vi "AnalogDemultiplexerV2_NI5771.vi"() -> ()   [LabVIEW 2012]
uses:
  <vilib>/Platform/TimedLoop/XDataNode/timing_clust.ctl
  <vilib>/Platform/TimedLoop/XDataNode/nitl_modes.ctl
  <vilib>/Platform/TimedLoop/XDataNode/wakeup.ctl
  <vilib>/rvi/FIFO/Fifo_Resource/nirvififoEmulationSetSize.vi
  <vilib>/rvi/DataTransferAndStorage/Container/Common/niFpgaContainerGetUniqueNameForEmu.vi
  <vilib>/rvi/eio/common/nirviEmuTemplateMethod_errors.vi
  <vilib>/rvi/Emulation/niFpgaSctlEmulationRegisterWithScheduler.vi
  <vilib>/rvi/errors/niFpgaSetErrorForExecOnDevCompSimple.vi
  <vilib>/rvi/eio/common/nirviEmuReportErrorAndStop.vi
  <vilib>/rvi/Emulation/niFpgaSctlEmulationFifoFullMgr.vi
  <vilib>/rvi/Emulation/niFpgaSctlEmulationResourceMgr.vi
  <vilib>/rvi/Emulation/niFpgaSctlEmulationScheduler.vi
  <vilib>/rvi/interface/RandomDataEmulation/nirviRandomDataFPGAFIFO.vi
  <vilib>/rvi/interface/RandomDataEmulation/niFpgaRandomDataHandleErrors.vi
  <vilib>/rvi/Emulation/niFpgaSctlEmulationGlobalWrite.vi
  <vilib>/Platform/TimedLoop/XDataNode/XDataNode.xnode
  <vilib>/rvi/DataTransferAndStorage/Container/XNode/niFpgaContainer.xnode
  <vilib>/rvi/FIFO/Fifo_Resource/nirvififoEmulationClear.vi
  <vilib>/eio/EIONode/EIONode.xnode
  <vilib>/rvi/FIFO/Fifo_Resource/nirvififoEmulationWrite.vi
  <vilib>/rvi/FIFO/Fifo_Resource/nirvififoEmulationRead.vi
  <vilib>/rvi/interface/RandomDataEmulation/nirviRandomDataFpgaReadWriteTemplate.vi
  <vilib>/Platform/TimedLoop/XDataNode/XDNodeRunTimeDep.lvlib
panel:
  in  "CutoffU8 Ch2":u8
  in  "CutoffU8 Ch1":u8
  out "ToHostA2FIFO Overflow":bool
  out "ToHostA1FIFO Overflow":bool
  out "Pixel counter A2":u32
  out "Pixel counter A1":u32
  out "InterloopFIFO Overflow":bool
  in  "BaselineU8 Ch2":u8
  in  "BaselineU8 Ch1":u8
  out "InterloopFIFO timeout":bool
  in  "Clear Interloop FIFO":bool
  out "Acquiring":bool
  in  "Wait for trigger":bool
  in  "Acquire":bool
  in  "Requested pixels A2":u32=100000 caption="Requested pixels"
  in  "Acquire continuously":bool=TRUE
  in  "Requested pixels A1":u32=100000 caption="Requested pixels"
  in  "Samples per pixel":u16=10000 caption="Samples per pixel Acq"
  out "IO Module\\AI Over Range":bool
  in  "User Command Commit":bool
  in  "User Command":u8
  out "User Command Idle":bool
  out "User Command Status":u8
  in  "User Data 0":u16
  in  "User Data 1":u8
  out "PLL Locked":bool
  out "User Error":bool
  out "Configured?":bool
  # "5771 IO module configuration"
  # "Analog demultiplexer V2"
  # "Acquisition control"
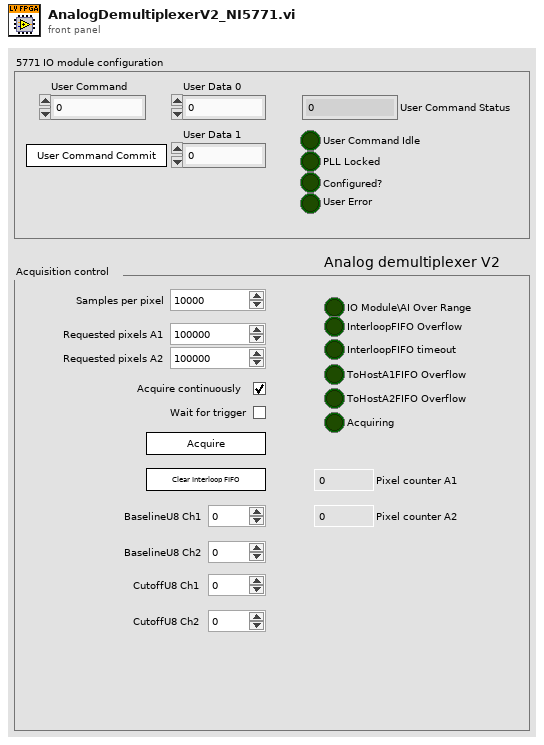
[diagram p1: front panel]
types:
  T1 = typedef "XDNodeRunTimeDep.lvlib/timing_clust.ctl" = cluster{"Expected End [f-1]":u64, "Actual End [f-1]":u64, "Finished Late? [f-1]":bool, "Expected End [i-1]":u64, "Actual End [i-1]":u64, "Finished Late? [i-1]":bool, "Expected Start [i]":u64, "Actual Start [i]":u64, "Expected Start [f]":u64, "Actual Start [f]":u64, "Source Name":string, "Structure Name":string, "Period":i64, "Deadline":i64, "Offset":i64, "Start":i64, "Priority":i32, "Timeout":i32, "Mode":T2, "Wakeup Reason":T3, "Error":errorcluster, "Source Type":string, "Secondary Source Type":string, "Global End Time":u64, "Global Start Time":u64, "Frame Duration":u64, "Iteration Duration":u64, "Assigned CPU":i32, "I/O Scan Engine Mode":u32}
  T2 = typedef "XDNodeRunTimeDep.lvlib/nitl_modes.ctl" = enum32{"No Change", "Process missed periods, maintain original phase", "Discard missed periods, maintain original phase", "Process missed periods, ignore original phase", "Discard missed periods, ignore original phase"}
  T3 = typedef "XDNodeRunTimeDep.lvlib/wakeup.ctl" = enum32{"Normal", "Aborted", "Asynchronous wakeup", "Timing source error", "Timed loop error", "Timeout"}
  T4 = cluster{"IO Module\\AI 0 Data N-7":u8, "IO Module\\AI 0 Data N-6":u8, "IO Module\\AI 0 Data N-5":u8, "IO Module\\AI 0 Data N-4":u8, "IO Module\\AI 0 Data N-3":u8, "IO Module\\AI 0 Data N-2":u8, "IO Module\\AI 0 Data N-1":u8, "IO Module\\AI 0 Data N":u8, "IO Module\\Synchronous Trigger Input":u8}
  T5 = cluster{"IO Module\\AI 1 Data N-7":u8, "IO Module\\AI 1 Data N-6":u8, "IO Module\\AI 1 Data N-5":u8, "IO Module\\AI 1 Data N-4":u8, "IO Module\\AI 1 Data N-3":u8, "IO Module\\AI 1 Data N-2":u8, "IO Module\\AI 1 Data N-1":u8, "IO Module\\AI 1 Data N":u8, "IO Module\\Synchronous Trigger Input":u8}
  T6 = cluster{"A1 Ch1":u32, "A1 Ch2":u32, "A2 Ch1":u32, "A2 Ch2":u32}
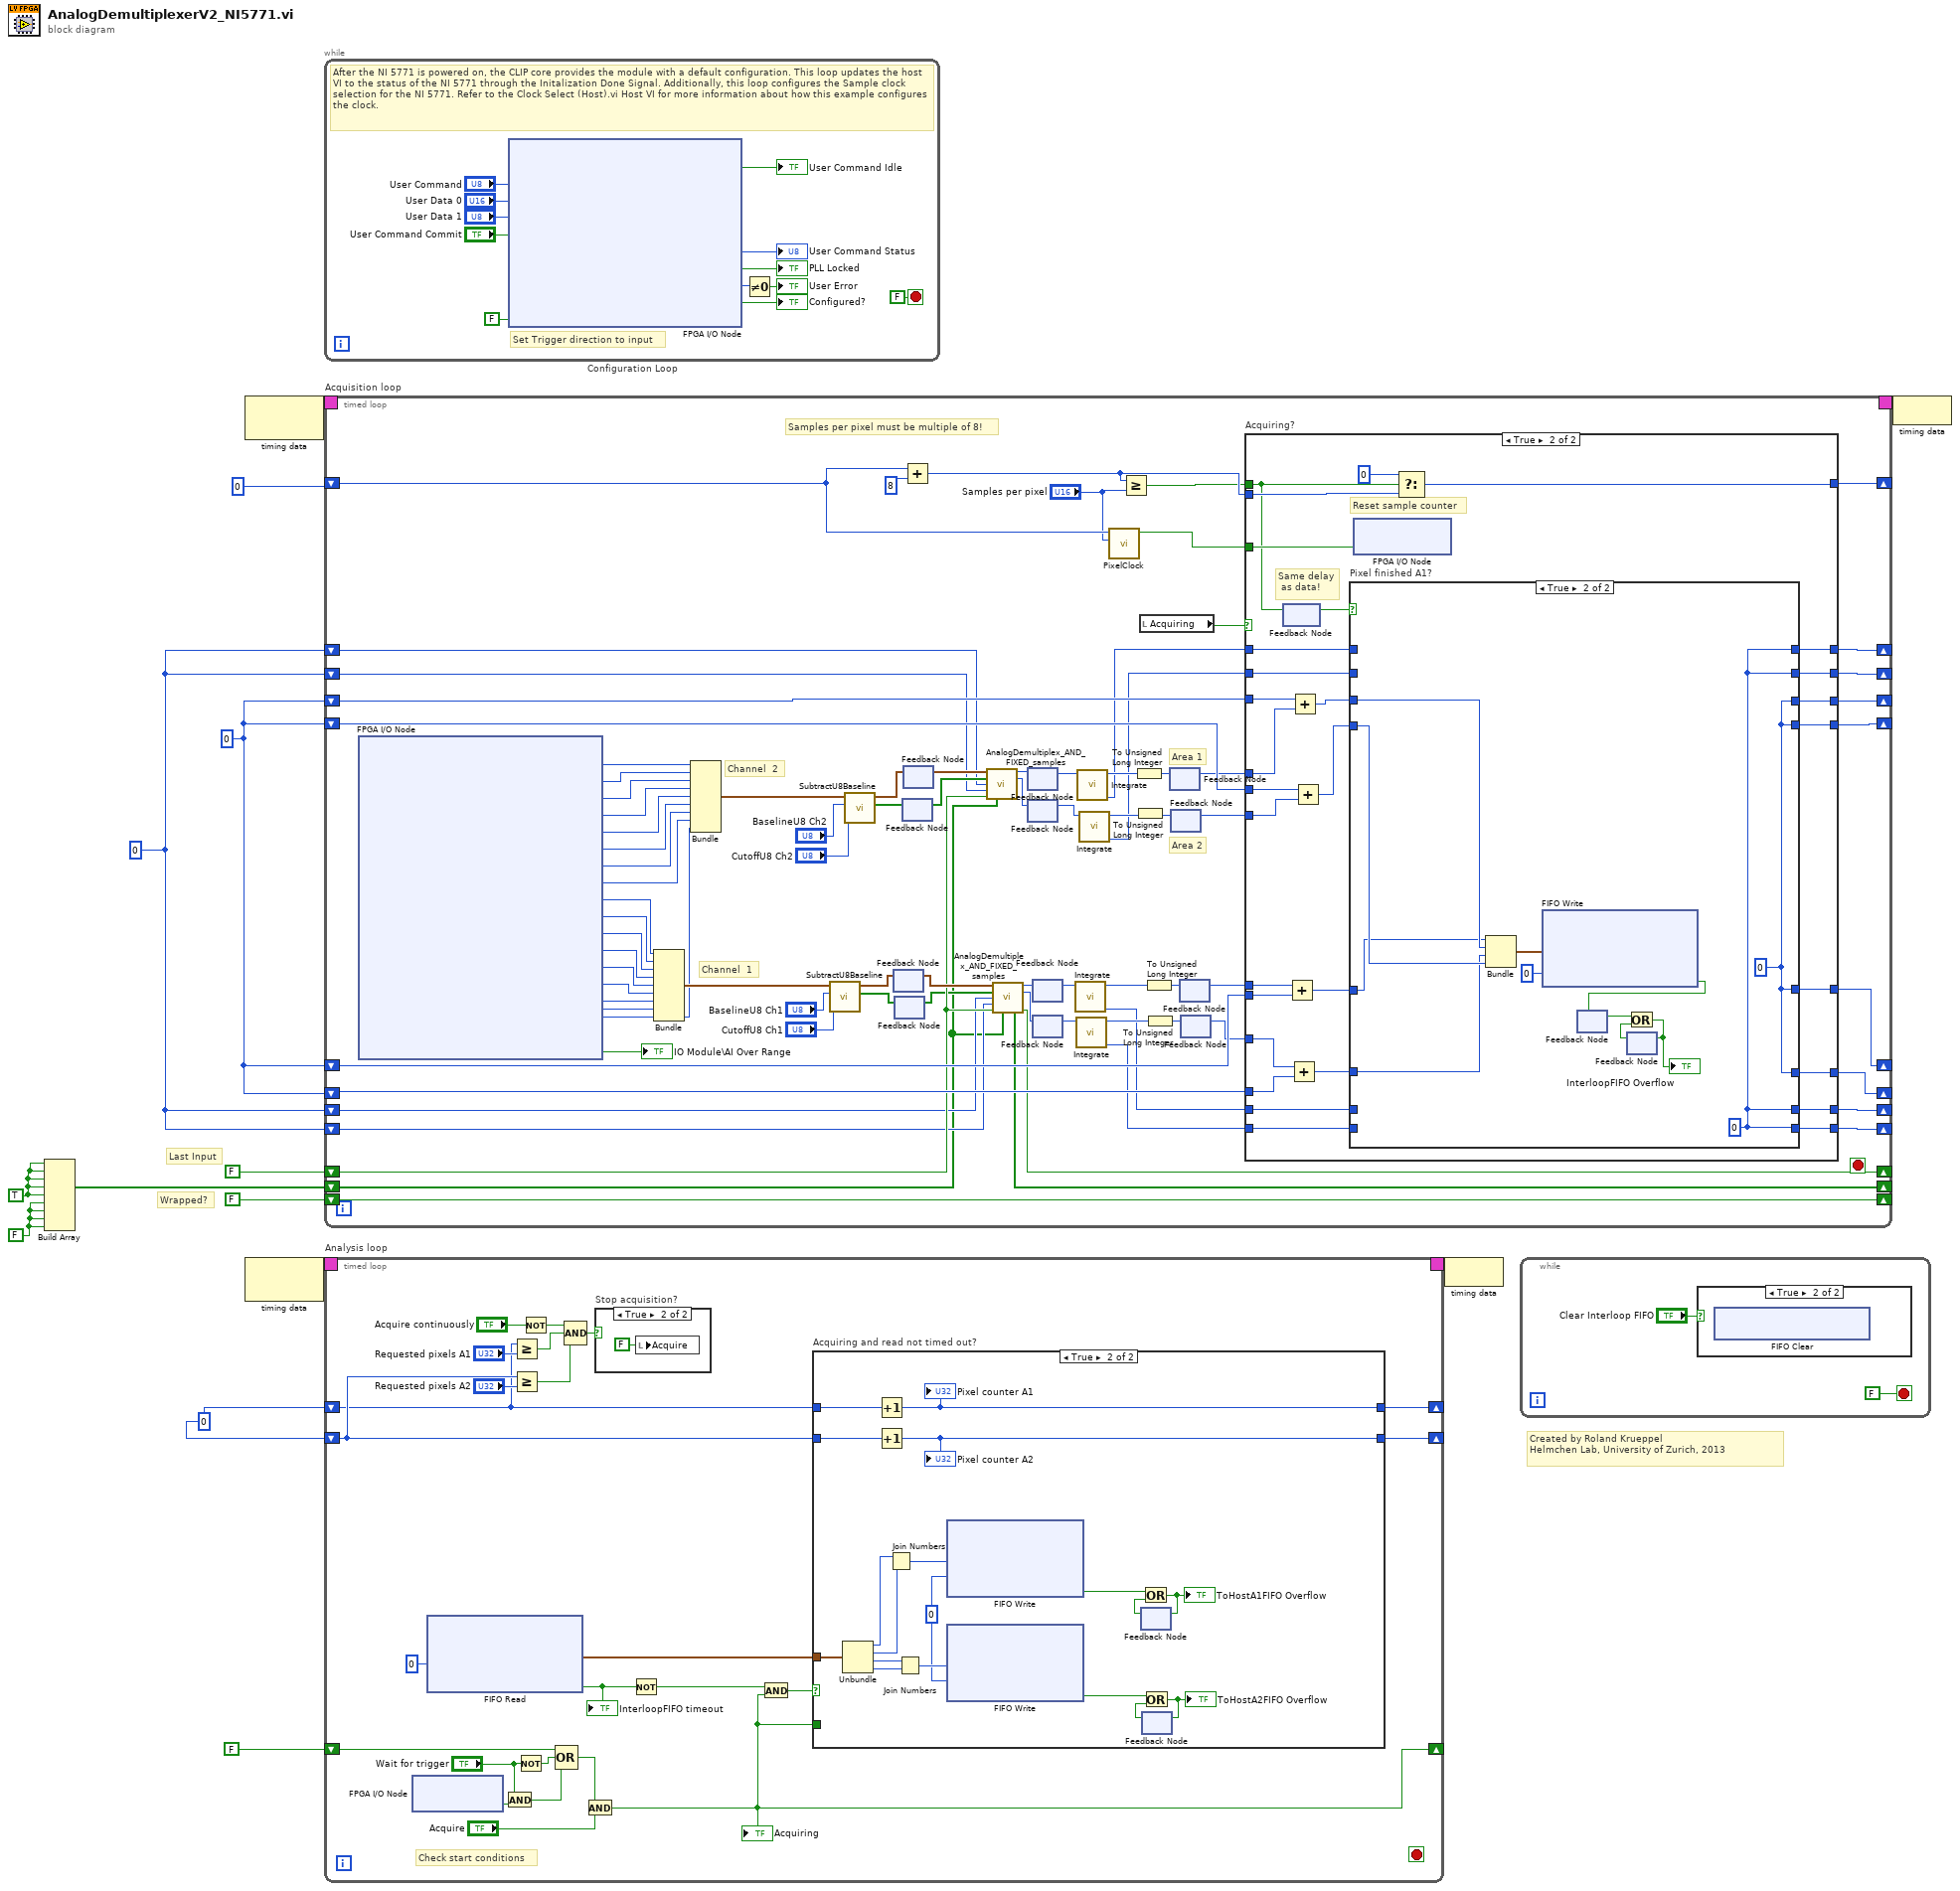
[diagram p0: block diagram]
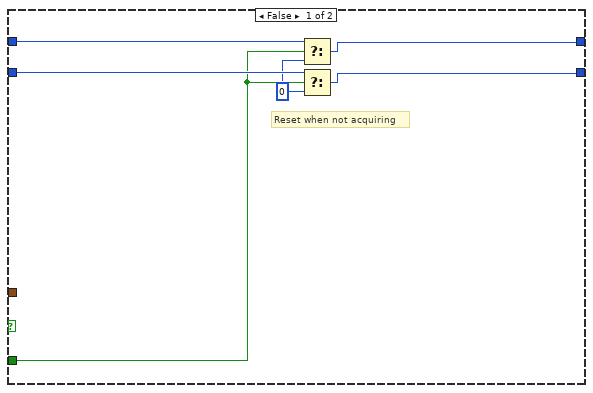
[diagram p3: hidden frame]
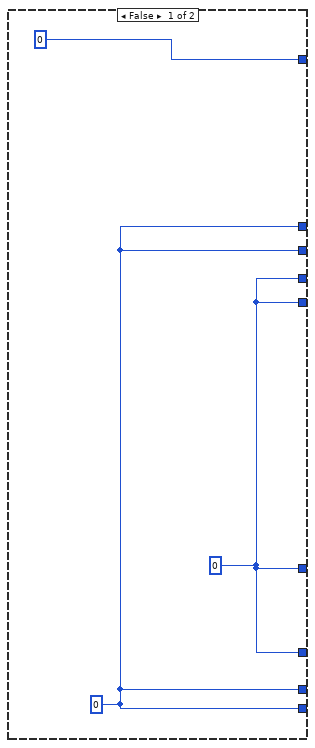
[diagram p5: hidden frame]
diagram:
  w1 = FALSE
  w2 = TRUE
  w4 = u8 0
  w6 = u32 0
  w9 = u32 0 ("Integrator out")
  # "Wrapped?"
  # "Last Input"
  # "Created by Roland Krueppel\nHelmchen Lab, University of Zurich, 2013"
  n1 = Build Array(w2, w2, w2, w2, w2, w1, w1, w1, w1) -> (w3:bool[])
  n2 = node-c288() -> (w14:T1)  [unwired: 1 in]
  n3 = node-c288() -> (w12:T1)  [unwired: 1 in]
  n4 = while "Configuration Loop" {
    stop <- FALSE stop-if-true
    # "Set Trigger direction to input"
    # "After the NI 5771 is powered on, the CLIP core provides the module with a default configuration. This loop updates the host VI to the status of the NI 5771 through the Initalization Done Signal. Additionally, this loop configures the Sample clock selection for the NI 5771. Refer to the Clock Select (Host).vi Host VI for more information about how this example configures the clock."
    n5 = xnode "FPGA I/O Node"("IO Module\\User Command"="User Command", "IO Module\\User Data 0"="User Data 0", "IO Module\\User Data 1"="User Data 1", "IO Module\\User Command Commit"="User Command Commit", "IO Module\\Trigger WE"=FALSE ("IO Module\\Trigger WE")) -> ("IO Module\\User Command Idle"=→"User Command Idle":bool, "IO Module\\User Command Status"=→"User Command Status":u8, "IO Module\\PLL Locked"=→"PLL Locked":bool, "IO Module\\User Error"=w19:u8, "IO Module\\Initialization Done"=→"Configured?":bool)  [unwired: 10 in, 10 out]
    n6 = Not Equal To 0?(x=w19) -> (x != 0?=→"User Error":bool)
  }
  n7 = timed-loop "Acquisition loop" {
    timing: w14 -> [_]
    timing-out: [_] -> w13
    shift-right: [w95] -> _
    shift-left: u16 0 -> [w86]
    shift-right: [w68] -> _
    shift-left: w6 -> [w77]
    shift-right: [w67] -> _
    shift-left: w6 -> [w76]
    shift-right: [w69] -> _
    shift-left: w6 -> [w78]
    shift-right: [w70] -> _
    shift-left: w6 -> [w79]
    shift-right: [w41] -> _
    shift-left: FALSE -> [w51]
    shift-right: [w56] -> _
    shift-left: FALSE -> [w56]
    shift-right: [w48] -> _
    shift-left: w4 -> [w30]
    shift-right: [w47] -> _
    shift-left: w4 -> [w29]
    shift-right: [w50] -> _
    shift-left: w4 -> [w31]
    shift-right: [w49] -> _
    shift-left: w4 -> [w32]
    shift-right: [w28] -> _
    shift-left: w3 -> [w27]
    stop <- _ stop-if-true
    # "Area 2"
    # "Area 1"
    # "Channel  2"
    # "Channel  1"
    # "Samples per pixel must be multiple of 8!"
    n8 = xnode "FPGA I/O Node"() -> ("IO Module\\AI 1 Data N-7"=w103:u8, "IO Module\\AI 1 Data N-6"=w102:u8, "IO Module\\AI 1 Data N-5"=w101:u8, "IO Module\\AI 1 Data N-4"=w100:u8, "IO Module\\AI 1 Data N-3"=w99:u8, "IO Module\\AI 1 Data N-2"=w98:u8, "IO Module\\AI 1 Data N-1"=w97:u8, "IO Module\\AI 1 Data N"=w96:u8, "IO Module\\AI 0 Data N-7"=w104:u8, "IO Module\\AI 0 Data N-6"=w105:u8, "IO Module\\AI 0 Data N-5"=w106:u8, "IO Module\\AI 0 Data N-4"=w107:u8, "IO Module\\AI 0 Data N-3"=w108:u8, "IO Module\\AI 0 Data N-2"=w109:u8, "IO Module\\AI 0 Data N-1"=w110:u8, "IO Module\\AI 0 Data N"=w111:u8, "IO Module\\Synchronous Trigger Input"=w66:u8, "IO Module\\AI Over Range"=→"IO Module\\AI Over Range":bool)  [unwired: 18 in, 18 out]
    n9 = Bundle("IO Module\\AI 0 Data N-7"=w104, "IO Module\\AI 0 Data N-6"=w105, "IO Module\\AI 0 Data N-5"=w106, "IO Module\\AI 0 Data N-4"=w107, "IO Module\\AI 0 Data N-3"=w108, "IO Module\\AI 0 Data N-2"=w109, "IO Module\\AI 0 Data N-1"=w110, "IO Module\\AI 0 Data N"=w111, "IO Module\\Synchronous Trigger Input"=w66) -> (w89:T4)  [unwired: 1 in]
    n10 = Bundle("IO Module\\AI 1 Data N-7"=w103, "IO Module\\AI 1 Data N-6"=w102, "IO Module\\AI 1 Data N-5"=w101, "IO Module\\AI 1 Data N-4"=w100, "IO Module\\AI 1 Data N-3"=w99, "IO Module\\AI 1 Data N-2"=w98, "IO Module\\AI 1 Data N-1"=w97, "IO Module\\AI 1 Data N"=w96, "IO Module\\Synchronous Trigger Input"=w66) -> (w91:T5)  [unwired: 1 in]
    n11 = call "SubtractU8Baseline.vi"("Cutoff U8"="CutoffU8 Ch1", "Baseline U8"="BaselineU8 Ch1", "Analog data cluster in"=w89) -> ("Over? Array"=w38:bool[], "Analog data cluster out"=w88:T4)  [unwired: 7 in]
    n12 = call "SubtractU8Baseline.vi"("Cutoff U8"="CutoffU8 Ch2", "Baseline U8"="BaselineU8 Ch2", "Analog data cluster in"=w91) -> ("Over? Array"=w40:bool[], "Analog data cluster out"=w90:T4)  [unwired: 7 in]
    n13 = feedback #1() -> (w65:T4)  [unwired: 1 in]
    n14 = feedback-in #1(w88) -> ()
    n15 = feedback #2() -> (w37:bool[])  [unwired: 1 in]
    n16 = feedback-in #2(w38) -> ()
    n17 = Add(x=w86, y=u16 8) -> (x+y=w93:u16)
    n18 = feedback #3() -> (w39:bool[])  [unwired: 1 in]
    n19 = feedback-in #3(w40) -> ()
    n20 = feedback-in #4(w90) -> ()
    n21 = feedback #4() -> (w57:T4)  [unwired: 1 in]
    n22 = call "AnalogDemultiplex_AND_FIXED_samples.vi"("Analog data cluster"=w57, "Over? Array"=w39, "Last Sample A1"=w31, "Last Sample A2"=w32, "Last? Input"=w51, "array in"=w27) -> ("Data A1 out"=w61:u64, "Data A2 out"=w59:u64)  [unwired: 6 in, 2 out]
    n23 = call "AnalogDemultiplex_AND_FIXED_samples.vi"("Analog data cluster"=w65, "Over? Array"=w37, "Last Sample A1"=w30, "Last Sample A2"=w29, "Last? Input"=w51, "array in"=w27) -> ("Data A1 out"=w64:u64, "Data A2 out"=w63:u64, "array out"=w28:bool[], "Last? Output"=w41:bool)  [unwired: 6 in]
    n24 = feedback-in #5(w61) -> ()
    n25 = feedback #5() -> (w60:u64)  [unwired: 1 in]
    n26 = feedback #6() -> (w58:u64)  [unwired: 1 in]
    n27 = feedback-in #6(w59) -> ()
    n28 = feedback #7() -> (w84:u64)  [unwired: 1 in]
    n29 = feedback-in #7(w64) -> ()
    n30 = feedback #8() -> (w62:u64)  [unwired: 1 in]
    n31 = feedback-in #8(w63) -> ()
    n32 = call "Integrate.vi"("New samples in"=w84) -> ("Next Sample"=w43:u8, "Sum out"=w44:u16)  [unwired: 9 in]
    n33 = call "Integrate.vi"("New samples in"=w62) -> ("Next Sample"=w42:u8, "Sum out"=w45:u16)  [unwired: 9 in]
    n34 = call "Integrate.vi"("New samples in"=w60) -> ("Next Sample"=w33:u8, "Sum out"=w36:u16)  [unwired: 9 in]
    n35 = call "Integrate.vi"("New samples in"=w58) -> ("Next Sample"=w34:u8, "Sum out"=w35:u16)  [unwired: 9 in]
    n36 = call "PixelClock.vi"("Samples per pixel"="Samples per pixel", "Sample counter"=w86) -> ("Pixel clock"=w85:bool)  [unwired: 9 in]
    n37 = Greater Or Equal?(x=w93, y="Samples per pixel") -> (x >= y?=w92:bool)
    n38 = To Unsigned Long Integer(number=w36) -> (unsigned 32bit integer=w83:u32)
    n39 = To Unsigned Long Integer(number=w35) -> (unsigned 32bit integer=w82:u32)
    n40 = local read "Acquiring"() -> (w71:bool)
    n41 = To Unsigned Long Integer(number=w44) -> (unsigned 32bit integer=w81:u32)
    n42 = To Unsigned Long Integer(number=w45) -> (unsigned 32bit integer=w80:u32)
    n43 = feedback #9() -> (w74:u32)  [unwired: 1 in]
    n44 = feedback-in #9(w83) -> ()
    n45 = feedback #10() -> (w73:u32)  [unwired: 1 in]
    n46 = feedback-in #10(w82) -> ()
    n47 = feedback #11() -> (w75:u32)  [unwired: 1 in]
    n48 = feedback-in #11(w81) -> ()
    n49 = feedback #12() -> (w72:u32)  [unwired: 1 in]
    n50 = feedback-in #12(w80) -> ()
    n51 = case "Acquiring?" shown="True" w71 {
      tunnel: [u16 0 ("t") w144] -> w95
      tunnel: w93 -> [_ w143]
      tunnel: w92 -> [_ w133]
      tunnel: w85 -> [_ w137]
      tunnel: w79 -> [_ w123]
      tunnel: w78 -> [_ w142]
      tunnel: w77 -> [_ w126]
      tunnel: w76 -> [_ w141]
      tunnel: w75 -> [_ w124]
      tunnel: w74 -> [_ w140]
      tunnel: w73 -> [_ w139]
      tunnel: w72 -> [_ w125]
      tunnel: [w114 w131] -> w70
      tunnel: [w114 w130] -> w69
      tunnel: [w114 w129] -> w68
      tunnel: [w114 w128] -> w67
      tunnel: [w112 w122] -> w50
      tunnel: [w112 w121] -> w49
      tunnel: [w112 w120] -> w48
      tunnel: [w112 w119] -> w47
      tunnel: w33 -> [_ w118]
      tunnel: w34 -> [_ w117]
      tunnel: w42 -> [_ w116]
      tunnel: w43 -> [_ w115]
      frame False {
        w112 = u8 0 ("t")
        w114 = u32 0
      }
      frame True {
        # "Same delay\n as data!"
        # "Reset sample counter"
        n52 = feedback #13() -> (w132:bool)  [unwired: 1 in]
        n53 = feedback-in #13(w133) -> ()
        n54 = Add(x=w124, y=w123) -> (x+y=w136:u32)
        n55 = Add(x=w125, y=w126) -> (x+y=w127:u32)
        n56 = Add(x=w142, y=w140) -> (x+y=w135:u32)
        n57 = Add(x=w141, y=w139) -> (x+y=w134:u32)
        n58 = case "Pixel finished A1?" shown="True" w132 {
          tunnel: w136 -> [w152 w154]
          tunnel: w135 -> [w151 w156]
          tunnel: w127 -> [w150 w153]
          tunnel: w134 -> [w149 w155]
          tunnel: [w152 w158] -> w131
          tunnel: [w151 w158] -> w130
          tunnel: [w150 w158] -> w129
          tunnel: [w149 w158] -> w128
          tunnel: [w148 w157] -> w122
          tunnel: [w147 w157] -> w121
          tunnel: [w145 w157] -> w120
          tunnel: [w146 w157] -> w119
          tunnel: w118 -> [w148 _]
          tunnel: w117 -> [w147 _]
          tunnel: w116 -> [w146 _]
          tunnel: w115 -> [w145 _]
          frame False {
          }
          frame True {
            w157 = u8 0
            w158 = u32 0
            n59 = Bundle(w154, w156, w153, w155) -> (w164:cluster{u32, u32, u32, u32})  [unwired: 1 in]
            n60 = xnode ("FIFO Write")("Element"=w164, "Timeout"=0) -> ("Timed Out?"=w159:bool)  [unwired: 1 in, 1 out]
            n61 = feedback #14() -> (w160:bool)  [unwired: 1 in]
            n62 = feedback-in #14(w159) -> ()
            n63 = feedback #15() -> (w161:bool)  [unwired: 1 in]
            n64 = Or(x=w160, y=w161) -> (x .or. y?=w162:bool)
            "InterloopFIFO Overflow" <- w162
            n65 = feedback-in #15(w162) -> ()
          }
        }
        n66 = xnode "FPGA I/O Node"("Pixel clock"=w137) -> ()  [unwired: 1 in, 1 out]
        n67 = Select(t=u16 0, s=w133, f=w143) -> (s? t:f=w144:u16)
      }
    }
  }
  n68 = timed-loop "Analysis loop" {
    timing: w12 -> [_]
    timing-out: [_] -> w11
    shift-right: [w167] -> _
    shift-left: FALSE -> [w177]
    shift-right: [w170] -> _
    shift-left: w9 -> [w171]
    shift-right: [w169] -> _
    shift-left: w9 -> [w172]
    stop <- _ stop-if-true
    # "Check start conditions"
    n69 = xnode "FPGA I/O Node"() -> ("TriggerIn"=w182:bool)  [unwired: 1 in, 1 out]
    n70 = xnode ("FIFO Read")("Timeout"=0) -> ("Element"=w168:T6, "Timed Out?"=w174:bool)  [unwired: 1 in, 1 out]
    "InterloopFIFO timeout" <- w174
    n71 = And(x="Wait for trigger", y=w182) -> (x .and. y?=w179:bool)
    n72 = Greater Or Equal?(x=w171, y="Requested pixels A1") -> (x >= y?=w185:bool)
    n73 = Greater Or Equal?(x=w172, y="Requested pixels A2") -> (x >= y?=w184:bool)
    n74 = Not(x="Wait for trigger") -> (.not. x?=w180:bool)
    n75 = Not(x="Acquire continuously") -> (.not. x?=w186:bool)
    n76 = Compound Arithmetic op=OR(w177, w180, w179) -> (w178:bool)
    n77 = Compound Arithmetic op=AND(w186, w185, w184) -> (w176:bool)
    n78 = And(x=w178, y="Acquire") -> (x .and. y?=w167:bool)
    "Acquiring" <- w167
    n79 = case "Stop acquisition?" shown="True" w176 {
      frame False {
      }
      frame True {
        n80 = local write "Acquire"(FALSE ("Acquire")) -> ()
      }
    }
    n81 = Not(x=w174) -> (.not. x?=w173:bool)
    n82 = And(x=w173, y=w167) -> (x .and. y?=w175:bool)
    n83 = case "Acquiring and read not timed out?" shown="True" w175 {
      tunnel: w172 -> [w194 w213]
      tunnel: w171 -> [w196 w214]
      tunnel: [w195 w211] -> w170
      tunnel: [w193 w212] -> w169
      tunnel: w168 -> [_ w210]
      tunnel: w167 -> [w192 _]
      frame False {
        w191 = u32 0 ("f")
        # "Reset when not acquiring"
        n84 = Select(t=w196, s=w192, f=w191) -> (s? t:f=w195:u32)
        n85 = Select(t=w194, s=w192, f=w191) -> (s? t:f=w193:u32)
      }
      frame True {
        w203 = 0 ("Timeout")
        n86 = Unbundle(w210) -> ("A1 Ch1"=w209:u32, "A1 Ch2"=w208:u32, "A2 Ch1"=w206:u32, "A2 Ch2"=w205:u32)
        n87 = Increment(x=w214) -> (x+1=w211:u32)
        "Pixel counter A1" <- w211
        n88 = Increment(x=w213) -> (x+1=w212:u32)
        "Pixel counter A2" <- w212
        n89 = Join Numbers(hi=w209, lo=w208) -> ((hi.lo)=w207:u64)
        n90 = Join Numbers(hi=w206, lo=w205) -> ((hi.lo)=w204:u64)
        n91 = xnode ("FIFO Write")("Element"=w207, "Timeout"=w203) -> ("Timed Out?"=w201:bool)  [unwired: 1 in, 1 out]
        n92 = xnode ("FIFO Write")("Element"=w204, "Timeout"=w203) -> ("Timed Out?"=w197:bool)  [unwired: 1 in, 1 out]
        n93 = feedback #16() -> (w200:bool)  [unwired: 1 in]
        n94 = Or(x=w201, y=w200) -> (x .or. y?=w202:bool)
        "ToHostA1FIFO Overflow" <- w202
        n95 = feedback-in #16(w202) -> ()
        n96 = feedback #17() -> (w198:bool)  [unwired: 1 in]
        n97 = Or(x=w197, y=w198) -> (x .or. y?=w199:bool)
        "ToHostA2FIFO Overflow" <- w199
        n98 = feedback-in #17(w199) -> ()
      }
    }
  }
  n99 = node-c288(w11) -> ()
  n100 = while {
    stop <- FALSE stop-if-true
    n101 = case shown="True" "Clear Interloop FIFO" {
      frame False {
      }
      frame True {
        n102 = xnode ("FIFO Clear")() -> ()  [unwired: 1 in, 1 out]
      }
    }
  }
  n103 = node-c288(w13) -> ()
